vi "UN_PSWRD.vi"() -> ()   [LabVIEW 2019]
panel:
  in  "PASSWORD 2":string
  in  "USERNAME 2":string
  in  "Password_List":string[](array[string])
  in  "Username_list":string[](array[string])
  in  "PASSWORD":string
  in  "USERNAME":string
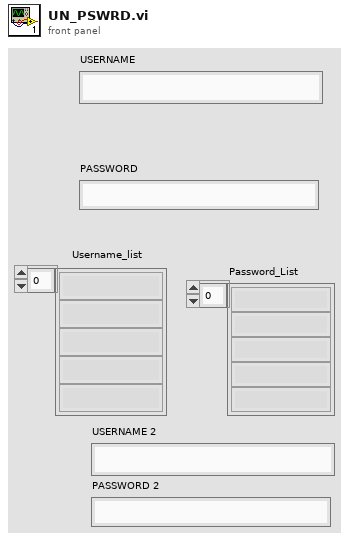
[diagram p1: front panel]
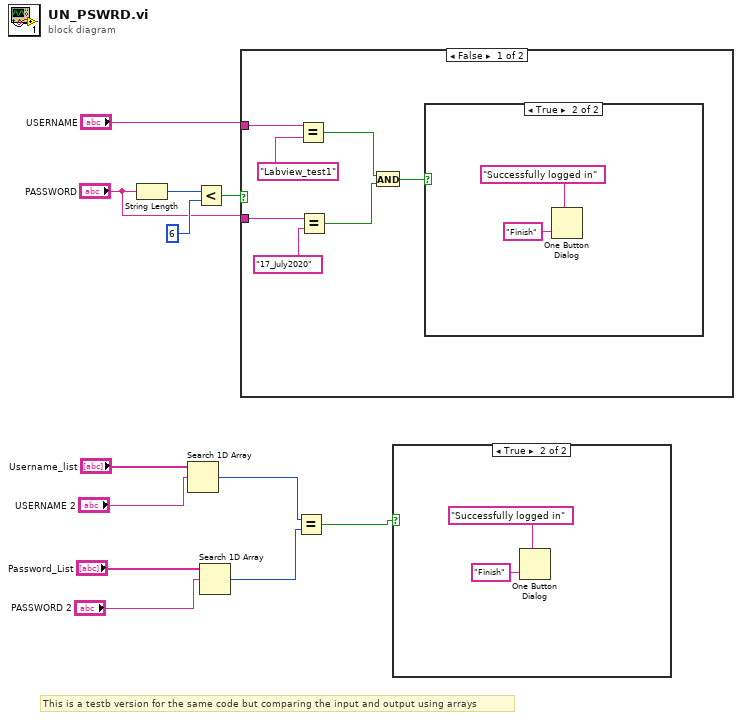
[diagram p0: block diagram]
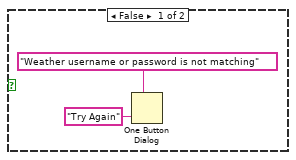
[diagram p2: hidden frame]
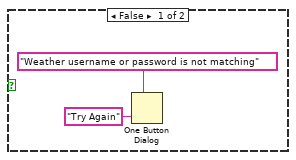
[diagram p3: hidden frame]
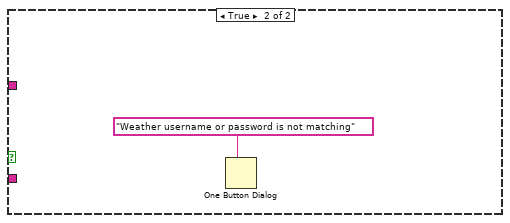
[diagram p4: hidden frame]
diagram:
  # "This is a testb version for the same code but comparing the input and output using arrays"
  n1 = String Length(string="PASSWORD") -> (length=w12:i32)
  n2 = Search 1D Array(1D array="Username_list", element="USERNAME 2") -> (index of element=w3:i32)  [unwired: 1 in]
  n3 = Less?(x=w12, y=6) -> (x < y?=w10:bool)
  n4 = Search 1D Array(1D array="Password_List", element="PASSWORD 2") -> (index of element=w2:i32)  [unwired: 1 in]
  n5 = case shown="False" w10 {
    tunnel: "USERNAME" -> [w19 _]
    tunnel: "PASSWORD" -> [w17 _]
    frame False {
      n6 = Equal?(x=w19, y="Labview_test1") -> (x = y?=w15:bool)
      n7 = Equal?(x=w17, y="17_July2020") -> (x = y?=w14:bool)
      n8 = And(x=w15, y=w14) -> (x .and. y?=w13:bool)
      n9 = case shown="True" w13 {
        frame False {
          n10 = One Button Dialog(message="Weather username or password is not matching", button name ("OK")="Try Again") -> ()  [unwired: 1 out]
        }
        frame True {
          n11 = One Button Dialog(message="Successfully logged in", button name ("OK")="Finish") -> ()  [unwired: 1 out]
        }
      }
    }
    frame True {
      n12 = One Button Dialog(message="Weather username or password is not matching") -> ()  [unwired: 1 in, 1 out]
    }
  }
  n13 = Equal?(x=w3, y=w2) -> (x = y?=w1:bool)
  n14 = case shown="True" w1 {
    frame False {
      n15 = One Button Dialog(message="Weather username or password is not matching", button name ("OK")="Try Again") -> ()  [unwired: 1 out]
    }
    frame True {
      n16 = One Button Dialog(message="Successfully logged in", button name ("OK")="Finish") -> ()  [unwired: 1 out]
    }
  }
